vi "Double FFT Mesurament (Max Bin detection - Control - Init Wave&Window - Snapshot - SingleFFT) RT Test.vi"() -> ()   [LabVIEW 2014]
uses:
  <vilib>/rvi/interface/nirviOpenFPGA/nirviOpenFPGA.xnode
  <vilib>/rvi/interface/nirviMethod/nirviMethod.xnode
  <vilib>/FPGAPlugInAG/Dynamic/niLvFpga_ConfigureFifo_Dynamic.vi
  <vilib>/rvi/errors/niLvFpgaMergeErrorWithErrorCode.vi
  <vilib>/FPGAPlugInAG/Dynamic/niLvFpga_StartFifo_Dynamic.vi
  <vilib>/FPGAPlugInAG/Dynamic/niLvFpga_Run_Dynamic.vi
  <vilib>/FPGAPlugInAG/Dynamic/niLvFpga_Abort_Dynamic.vi
  <vilib>/rvi/interface/nirviCloseFPGA/nirviCloseFPGA.xnode
  <vilib>/rvi/interface/nirviReadWriteControl/nirviReadWriteControl.xnode
  <vilib>/rvi/interface/Simulation/niFpgaSimulationCallBeginRW.vi
  <vilib>/rvi/errors/niLvFpgaAdjustHostInterfaceError.vi
  <vilib>/FPGAPlugInAG/Dynamic/niLvFpga_ReadFifo_Dynamic.vi
  <vilib>/Platform/TimedLoop/XDataNode/XDataNode.xnode
  <vilib>/Platform/TimedLoop/XDataNode/nitl_modes.ctl
  <vilib>/Platform/TimedLoop/XDataNode/XDNodeRunTimeDep.lvlib
  <vilib>/Platform/TimedLoop/XDataNode/wakeup.ctl
  <vilib>/Platform/TimedLoop/XDataNode/timing_clust.ctl
  <vilib>/FPGAPlugInAG/Dynamic/niLvFpga_Reset_Dynamic.vi
  FPGA Bitfiles/LaserDistanceSen_FPGATarget_DoubleFFTMesuram_y+9DFWHgHA4.lvbitx
  FPGA Target/Test VIs/Double FFT Mesurament (Max Bin detection - Control - Init Wave&Window - Snapshot - SingleFFT) test.vi
  NiFpgaLv.dll
  <vilib>/Utility/error.llb/Error Cluster From Error Code.vi
  <vilib>/FPGAPlugInAG/Dynamic/niLvFpga_Close_Dynamic.vi
  <vilib>/FPGAPlugInAG/sbRIO-9636/niLvFpga_Open_sbRIO-9636.vi
  <vilib>/rvi/interface/common/dynamic/niFpgaDynamicAddResources.vi
panel:
  out "Elements Remaining FFT":u32
  out "Elements Remaining Signal":u32
  out "Elements Remaining Signal":u32
  out "Elements Remaining FFT":u32
  out "FFT (bin)":dbl[](graph)
  out "Signal (t)":waveform(dbl)(graph)
  in  "Snapshot":bool
  in  "Windowing":T1(ring)
  in  "first bin":i32=10
  in  "last bin":i32=255
  in  "lower limit 2":u32(slide)=677 scale=625.0..738.0
  in  "lower limit 1":u32(slide)=59 scale=0.0..113.0
  out "Detected Frequency Tone - (Hz)":dbl
  in  "stop":bool
  out "Max Bin":i32
  out "Max Amp":dbl format="%.2f"
  out "Prev Bin":i32
  out "Next Bin":i32
  out "Prev Amp":dbl format="%.2f"
  out "Next Amp":dbl format="%.2f"
  out "Interpolated Bin":dbl
  in  "Interpolation Method":T2(ring)=enum."Jain"
  # "WARNING:\nOnce pressed wait untill the end of operation"
  # "ONLINE parameter"
  # "OFFLINE parameters"
  # "Max Detection FFT bin range"
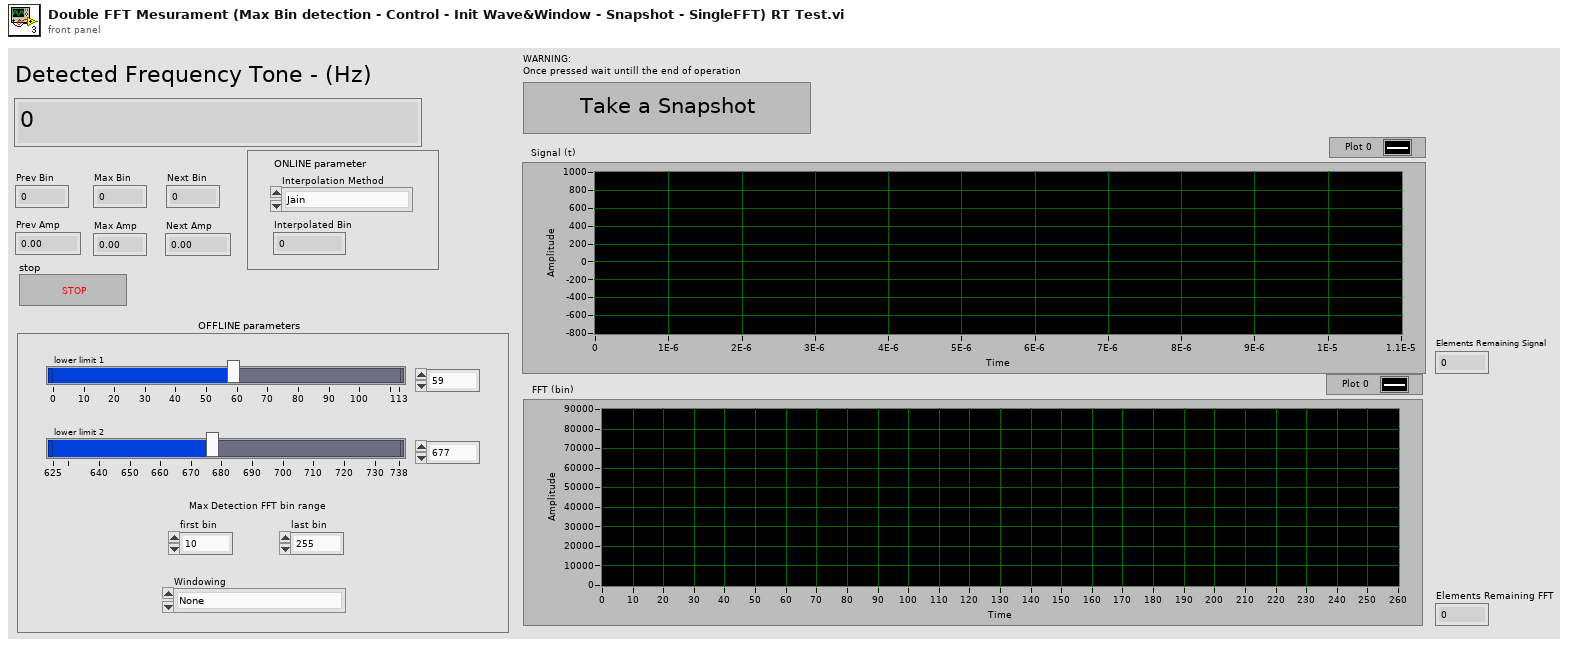
[diagram p1: front panel]
types:
  T1 = enum16{"None", "Hanning", "Hamming", "Blackman", "Blackman-Harris"}
  T2 = enum16{"Quadratic", "McLeodd", "Barycentric", "Jain"}
  T3 = typedef "XDNodeRunTimeDep.lvlib/timing_clust.ctl" = cluster{"Expected End [f-1]":u64, "Actual End [f-1]":u64, "Finished Late? [f-1]":bool, "Expected End [i-1]":u64, "Actual End [i-1]":u64, "Finished Late? [i-1]":bool, "Expected Start [i]":u64, "Actual Start [i]":u64, "Expected Start [f]":u64, "Actual Start [f]":u64, "Source Name":string, "Structure Name":string, "Period":i64, "Deadline":i64, "Offset":i64, "Start":i64, "Priority":i32, "Timeout":i32, "Mode":T4, "Wakeup Reason":T5, "Error":errorcluster, "Source Type":string, "Secondary Source Type":string, "Global End Time":u64, "Global Start Time":u64, "Frame Duration":u64, "Iteration Duration":u64, "Assigned CPU":i32, "I/O Scan Engine Mode":u32}
  T4 = typedef "XDNodeRunTimeDep.lvlib/nitl_modes.ctl" = enum32{"No Change", "Process missed periods, maintain original phase", "Discard missed periods, maintain original phase", "Process missed periods, ignore original phase", "Discard missed periods, ignore original phase"}
  T5 = typedef "XDNodeRunTimeDep.lvlib/wakeup.ctl" = enum32{"Normal", "Aborted", "Asynchronous wakeup", "Timing source error", "Timed loop error", "Timeout"}
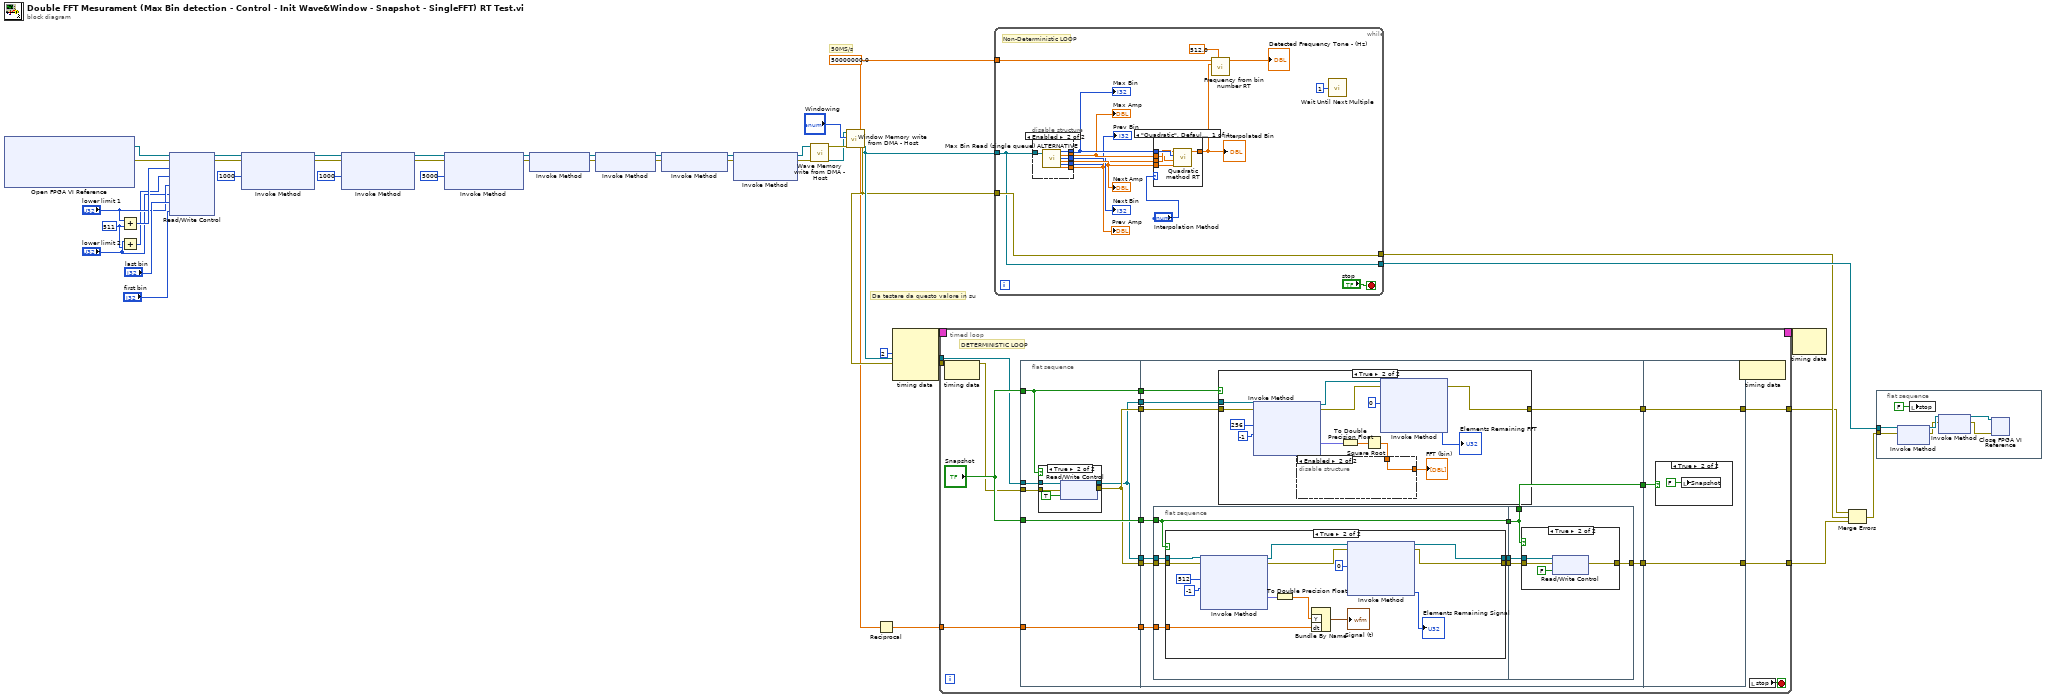
[diagram p0: block diagram]
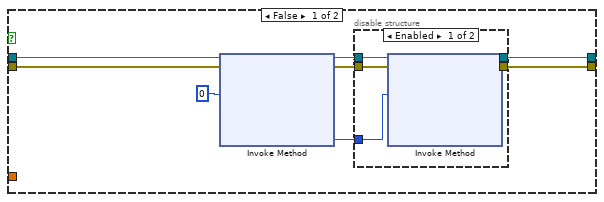
[diagram p3: hidden frame]
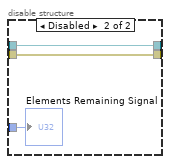
[diagram p4: hidden frame]
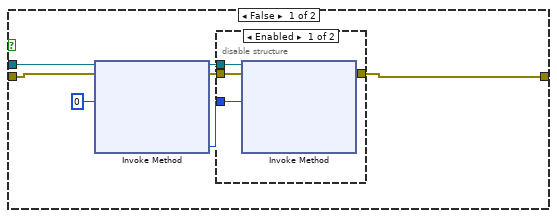
[diagram p6: hidden frame]
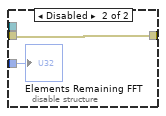
[diagram p7: hidden frame]
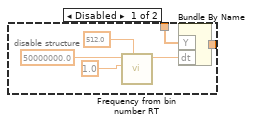
[diagram p8: hidden frame]
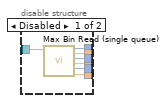
[diagram p10: hidden frame]
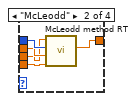
[diagram p11: hidden frame]
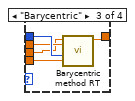
[diagram p12: hidden frame]
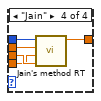
[diagram p13: hidden frame]
diagram:
  w37 = u32 511 ("y")
  w14 = 50000000.0 ("Sample Rate (S/s)")
  # "Da testare da questo valore in su"
  # "50MS/s"
  n1 = xnode "Open FPGA VI Reference"() -> ("FPGA VI Reference Out"=w36:refnum<k20>, "error out"=w35:errorcluster)  [unwired: 2 in]
  n2 = Add(x="lower limit 1", y=w37) -> (x+y=w41:u32)
  n3 = Add(x="lower limit 2", y=w37) -> (x+y=w39:u32)
  n4 = xnode "Read/Write Control"("FPGA VI Reference In"=w36, "error in"=w35, "upper limit 1"=w41, "upper limit 2"=w39, "lower limit 1"="lower limit 1", "lower limit 2"="lower limit 2", "last bin"="last bin", "first bin"="first bin") -> ("FPGA VI Reference Out"=w30:refnum<k20>, "error out"=w29:errorcluster)
  n5 = xnode "Invoke Method"("FPGA VI Reference In"=w30, "error in"=w29, "Requested Depth"=u32 1000) -> ("FPGA VI Reference Out"=w28:refnum<k20>, "error out"=w27:errorcluster)  [unwired: 1 out]
  n6 = xnode "Invoke Method"("FPGA VI Reference In"=w28, "error in"=w27, "Requested Depth"=u32 1000) -> ("FPGA VI Reference Out"=w26:refnum<k20>, "error out"=w25:errorcluster)  [unwired: 1 out]
  n7 = xnode "Invoke Method"("FPGA VI Reference In"=w26, "error in"=w25, "Requested Depth"=u32 5000) -> ("FPGA VI Reference Out"=w8:refnum<k20>, "error out"=w9:errorcluster)  [unwired: 1 out]
  n8 = xnode "Invoke Method"("FPGA VI Reference In"=w8, "error in"=w9) -> ("FPGA VI Reference Out"=w19:refnum<k20>, "error out"=w18:errorcluster)
  n9 = xnode "Invoke Method"("FPGA VI Reference In"=w19, "error in"=w18) -> ("FPGA VI Reference Out"=w21:refnum<k20>, "error out"=w20:errorcluster)
  n10 = xnode "Invoke Method"("FPGA VI Reference In"=w21, "error in"=w20) -> ("FPGA VI Reference Out"=w6:refnum<k20>, "error out"=w7:errorcluster)
  n11 = xnode "Invoke Method"("FPGA VI Reference In"=w6, "error in"=w7) -> ("FPGA VI Reference Out"=w13:refnum<k20>, "error out"=w12:errorcluster)  [unwired: 1 in]
  n12 = call "Wave Memory write from DMA - Host.vi"("error in"=w12, "FPGA VI Reference In"=w13) -> ("FPGA VI Reference Out"=w10:refnum<k20>, "error out"=w11:errorcluster)  [unwired: 7 in, 1 out]
  n13 = call "Window Memory write from DMA - Host.vi"("error in"=w11, "Enum"="Windowing", "FPGA VI Reference In"=w10) -> ("FPGA VI Reference Out"=w32:refnum<k20>, "error out"=w31:errorcluster)  [unwired: 5 in, 2 out]
  n14 = Reciprocal(x=w14) -> (1/x=w15:dbl)
  n15 = node-c288(i64 2 ("Period")) -> (w3:T3)  [unwired: 3 in]
  n16 = timed-loop {
    tunnel: w32 -> [w54]
    tunnel: w31 -> [w55]
    tunnel: [w57] -> w4
    tunnel: w15 -> [w59]
    tunnel: [w58] -> w5
    timing: w3 -> [_]
    timing-out: [_] -> w2
    stop <- w60 stop-if-true
    # "DETERMINISTIC LOOP"
    n17 = node-c288() -> ()  [unwired: 1 in, 1 out]
    n18 = flat-sequence {
      tunnel: w54 -> [w65]
      tunnel: w55 -> [w66]
      tunnel: "Snapshot" -> [w63]
      tunnel: "Snapshot" -> [w68]
      tunnel: w59 -> [w69]
      tunnel: [w67] -> w53
      tunnel: [w69] -> w52
      tunnel: [w68] -> w51
      tunnel: [w63] -> w50
      tunnel: [w67] -> w49
      tunnel: [w64] -> w48
      tunnel: [w64] -> w47
      tunnel: w53 -> [w85]
      tunnel: w52 -> [w84]
      tunnel: w51 -> [w77]
      tunnel: w50 -> [w81]
      tunnel: w49 -> [w80]
      tunnel: w48 -> [w79]
      tunnel: w47 -> [w86]
      tunnel: [w83] -> w46
      tunnel: [w82] -> w45
      tunnel: [w78] -> w44
      tunnel: [w169] -> w57
      tunnel: [w170] -> w58
      tunnel: w46 -> [w170]
      tunnel: w45 -> [w169]
      tunnel: w44 -> [w168]
      frame #0 {
        n19 = case shown="True" w63 {
          tunnel: [w70 w75] -> w67
          tunnel: w66 -> [w70 w74]
          tunnel: w65 -> [w71 w73]
          tunnel: [w71 w72] -> w64
          frame False {
          }
          frame True {
            n20 = xnode "Read/Write Control"("FPGA VI Reference In"=w73, "error in"=w74, "snapshot"=TRUE) -> ("FPGA VI Reference Out"=w72:refnum<k20>, "error out"=w75:errorcluster)
          }
        }
      }
      frame #1 {
        n21 = flat-sequence {
          tunnel: w86 -> [w95]
          tunnel: w85 -> [w94]
          tunnel: w84 -> [w93]
          tunnel: w77 -> [w90]
          tunnel: [w92] -> w89
          tunnel: [w91] -> w88
          tunnel: [w90] -> w87
          tunnel: [w127] -> w82
          tunnel: w89 -> [w129]
          tunnel: w88 -> [w128]
          tunnel: w87 -> [w126]
          tunnel: [w126] -> w78
          frame #0 {
            n22 = case shown="True" w90 {
              tunnel: w95 -> [w102 w125]
              tunnel: w94 -> [w100 w124]
              tunnel: [w99 w114] -> w91
              tunnel: w93 -> [_ w120]
              tunnel: [w96 w113] -> w92
              frame False {
                n23 = xnode "Invoke Method"("FPGA VI Reference In"=w102, "error in"=w100, "Number of Elements"=u32 0) -> ("FPGA VI Reference Out"=w98:refnum<k20>, "error out"=w97:errorcluster, "Elements Remaining"=w101:u32)  [unwired: 1 in, 1 out]
                n24 = disable-structure shown="Enabled" {
                  disable-tunnel: w101 -> [w108 w111]
                  disable-tunnel: [w107 w110] -> w99
                  disable-tunnel: w98 -> [w106 w109]
                  disable-tunnel: w97 -> [w105 w110]
                  disable-tunnel: [w104 w109] -> w96
                  frame Enabled {
                    n25 = xnode "Invoke Method"("FPGA VI Reference In"=w106, "error in"=w105, "Number of Elements"=w108) -> ("FPGA VI Reference Out"=w104:refnum<k20>, "error out"=w107:errorcluster)  [unwired: 1 in, 2 out]
                  }
                  frame Disabled {
                    "Elements Remaining Signal" <- w111
                  }
                }
              }
              frame True {
                n26 = xnode "Invoke Method"("FPGA VI Reference In"=w125, "error in"=w124, "Number of Elements"=u32 512, "Timeout (ms)"=-1) -> ("FPGA VI Reference Out"=w116:refnum<k20>, "error out"=w115:errorcluster, "Data"=w119:fxp<+/-,12,12>[])  [unwired: 1 out]
                n27 = To Double Precision Float(number=w119) -> (double precision float=w118:dbl[])
                n28 = Bundle By Name("Y"=w118, "dt"=w120) -> (→"Signal (t)":waveform(dbl))  [unwired: 1 in]
                n29 = xnode "Invoke Method"("FPGA VI Reference In"=w116, "error in"=w115, "Number of Elements"=u32 0) -> ("FPGA VI Reference Out"=w113:refnum<k20>, "error out"=w114:errorcluster, "Elements Remaining"=→"Elements Remaining Signal":u32)  [unwired: 1 in, 1 out]
              }
            }
          }
          frame #1 {
            n30 = case shown="True" w126 {
              tunnel: [w130 w132] -> w127
              tunnel: w129 -> [_ w133]
              tunnel: w128 -> [w130 w131]
              frame False {
              }
              frame True {
                n31 = xnode "Read/Write Control"("FPGA VI Reference In"=w133, "error in"=w131, "snapshot"=FALSE) -> ("error out"=w132:errorcluster)  [unwired: 1 out]
              }
            }
          }
        }
        n32 = case shown="True" w81 {
          tunnel: w79 -> [w140 w153]
          tunnel: w80 -> [w137 w154]
          tunnel: [w136 w152] -> w83
          frame False {
            n33 = xnode "Invoke Method"("FPGA VI Reference In"=w140, "error in"=w137, "Number of Elements"=u32 0) -> ("FPGA VI Reference Out"=w138:refnum<k20>, "error out"=w135:errorcluster, "Elements Remaining"=w139:u32)  [unwired: 1 in, 1 out]
            n34 = disable-structure shown="Enabled" {
              disable-tunnel: w139 -> [w145 w147]
              disable-tunnel: w138 -> [w144 _]
              disable-tunnel: [w143 w146] -> w136
              disable-tunnel: w135 -> [w142 w146]
              frame Enabled {
                n35 = xnode "Invoke Method"("FPGA VI Reference In"=w144, "error in"=w142, "Number of Elements"=w145) -> ("error out"=w143:errorcluster)  [unwired: 1 in, 3 out]
              }
              frame Disabled {
                "Elements Remaining FFT" <- w147
              }
            }
          }
          frame True {
            n36 = xnode "Invoke Method"("FPGA VI Reference In"=w153, "error in"=w154, "Number of Elements"=u32 256, "Timeout (ms)"=-1) -> ("FPGA VI Reference Out"=w150:refnum<k20>, "error out"=w151:errorcluster, "Data"=w158:fxp<+,44,44>[])  [unwired: 1 out]
            n37 = To Double Precision Float(number=w158) -> (double precision float=w157:dbl[])
            n38 = Square Root(x=w157) -> (sqrt(x)=w156:dbl[])
            n39 = disable-structure shown="Enabled" {
              disable-tunnel: w156 -> [w162 w167]
              disable-tunnel: [w161 w167] -> w155
              frame Disabled {
                n40 = call "Frequency from bin number RT.vi"("FFT size"=512.0, "Bin number"=1.0, "Sample Rate (S/s)"=50000000.0) -> ("Detected Frequency (Hz)"=w163:dbl)  [unwired: 8 in]
                n41 = Bundle By Name("Y"=w162, "dt"=w163) -> (w161:waveform(dbl))  [unwired: 1 in]
              }
              frame Enabled {
              }
            }
            "FFT (bin)" <- w155
            n42 = xnode "Invoke Method"("FPGA VI Reference In"=w150, "error in"=w151, "Number of Elements"=u32 0) -> ("error out"=w152:errorcluster, "Elements Remaining"=→"Elements Remaining FFT":u32)  [unwired: 1 in, 2 out]
          }
        }
      }
      frame #2 {
        n43 = case shown="True" w168 {
          frame False {
          }
          frame True {
            n44 = local write "Snapshot"(FALSE ("Snapshot")) -> ()
          }
        }
      }
    }
    n45 = node-c288() -> ()  [unwired: 1 in, 1 out]
    n46 = local read "stop"() -> (w60:bool)
  }
  n47 = while {
    tunnel: w14 -> [w185]
    tunnel: w32 -> [w183]
    tunnel: w31 -> [w184]
    tunnel: [w183] -> w34
    tunnel: [w184] -> w17
    stop <- "stop" stop-if-true
    # "Non-Deterministic LOOP"
    n48 = disable-structure shown="Enabled" {
      disable-tunnel: w183 -> [w193 w200]
      disable-tunnel: [w192 w199] -> w179
      disable-tunnel: [w191 w198] -> w178
      disable-tunnel: [w190 w196] -> w177
      disable-tunnel: [w189 w194] -> w176
      disable-tunnel: [w188 w195] -> w175
      disable-tunnel: [w187 w197] -> w174
      frame Disabled {
        n49 = call "Max Bin Read (single queue).vi"("FPGA VI Reference In"=w193) -> ("Max Bin"=w192:i32, "Max Amp"=w191:dbl, "Next Bin"=w187:i32, "Next Amp"=w190:dbl, "Prev Bin"=w188:i32, "Prev Amp"=w189:dbl)  [unwired: 13 in]
      }
      frame Enabled {
        n50 = call "Max Bin Read (single queue) ALTERNATIVE.vi"("FPGA VI Reference In"=w200) -> ("Max Bin"=w199:i32, "Max Amp"=w198:dbl, "Next Bin"=w197:i32, "Next Amp"=w196:dbl, "Prev Bin"=w195:i32, "Prev Amp"=w194:dbl)  [unwired: 13 in]
      }
    }
    "Max Bin" <- w179
    "Max Amp" <- w178
    "Prev Bin" <- w175
    "Next Bin" <- w174
    "Prev Amp" <- w176
    "Next Amp" <- w177
    n51 = case shown="\"Quadratic\", Default" "Interpolation Method" {
      tunnel: w179 -> [w204 w209 w214 w219]
      tunnel: w178 -> [w201 w208 w213 w218]
      tunnel: w176 -> [w202 w207 w212 w217]
      tunnel: w177 -> [w203 w206 w211 w216]
      tunnel: [w205 w210 w215 w220] -> w180
      frame "Quadratic", Default {
        n52 = call "Quadratic method RT.vi"("Next Amplitude"=w203, "Max Amplitude"=w201, "Max bin"=w204, "Prev Amplitude"=w202) -> ("Bin"=w205:dbl)  [unwired: 7 in]
      }
      frame "McLeodd" {
        n53 = call "McLeodd method RT.vi"("Next Amp"=w206, "Max Amp"=w208, "Max Bin"=w209, "Prev Amp"=w207) -> ("Bin"=w210:dbl)  [unwired: 7 in]
      }
      frame "Barycentric" {
        n54 = call "Barycentric method RT.vi"("Next Amp"=w211, "Max Bin"=w214, "Max Amp"=w213, "Prev Amp"=w212) -> ("Bin"=w215:dbl)  [unwired: 7 in]
      }
      frame "Jain" {
        n55 = call "Jain's method RT.vi"("Prev Amp"=w217, "Next Amp"=w216, "Max Amp"=w218, "Max Bin"=w219) -> ("Bin"=w220:dbl)  [unwired: 7 in]
      }
    }
    "Interpolated Bin" <- w180
    n56 = call "Frequency from bin number RT.vi"("FFT size"=512.0, "Bin number"=w180, "Sample Rate (S/s)"=w185) -> ("Detected Frequency (Hz)"=→"Detected Frequency Tone - (Hz)":dbl)  [unwired: 8 in]
    n57 = call "Wait Until Next Multiple"("Count(mSec)"=u32 1 ("Count(uSec)")) -> ()  [unwired: 1 out]
  }
  n58 = node-c288(w2) -> ()  [unwired: 1 out]
  n59 = Merge Errors(w5, w17, w4) -> (w16:errorcluster)
  n60 = flat-sequence {
    tunnel: w34 -> [w227]
    tunnel: w16 -> [w226]
    frame #0 {
      n61 = xnode "Invoke Method"("FPGA VI Reference In"=w227, "error in"=w226) -> ("FPGA VI Reference Out"=w222:refnum<k20>, "error out"=w221:errorcluster)
      n62 = local write "stop"(FALSE ("stop")) -> ()
      n63 = xnode "Invoke Method"("FPGA VI Reference In"=w222, "error in"=w221) -> ("FPGA VI Reference Out"=w223:refnum<k20>, "error out"=w224:errorcluster)
      n64 = xnode "Close FPGA VI Reference"("FPGA VI Reference In"=w223, "error in"=w224) -> ()  [unwired: 1 out]
    }
  }
